vi "Trade.vi"(11 "buffer.in":u64[](array[numeric])=[0, 0, 0, 0, 0, 0, 0, 0, 0]) -> (3 "OrderBook.Command":T1)   [LabVIEW 2020]
doc: "Cboe PITCH Trade (0x2A long, 0x2B short, 0x30 expanded) -> orderbook.command: type Trade (enum value 10, add Trade=10 and Unsupported=11 to orderbook.command.type.ctl), orderId, side, quantity, symbol (8 chars, space padded), price, nanoseconds. Short price keeps 2 implied decimals."
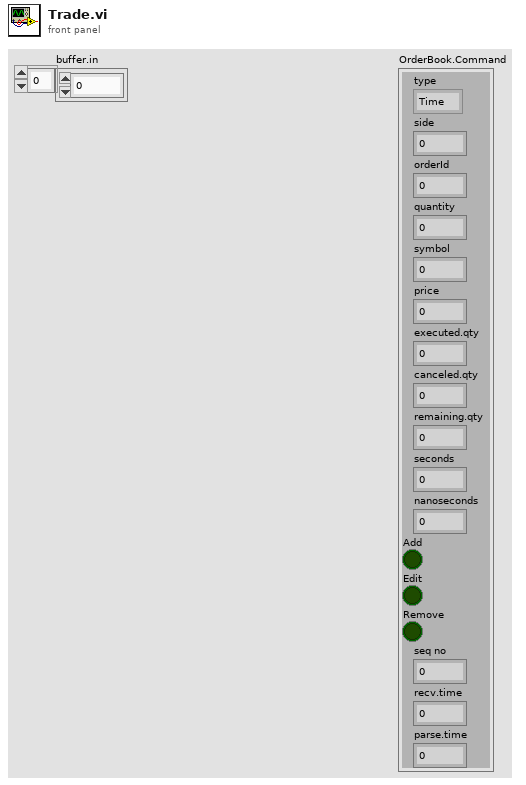
[diagram p1: front panel]
types:
  T1 = cluster{"type":enum8{"Time", "AddOrder", "OrderExecuted", "OrderExecutedAtPrice", "ReduceSize", "ModifyOrder", "DeleteOrder", "Get.Everything", "Get.All.Orders", "Get.Top", "Trade", "Unsupported"}, "side":u8, "orderId ":u64, "quantity":u32, "symbol":u64, "price":u64, "executed.qty":u32, "canceled.qty":u32, "remaining.qty":u32, "seconds":u64, "nanoseconds":u64, "Add":bool, "Edit":bool, "Remove":bool, "seq no":u32, "recv.time":u64, "parse.time":u64}
  T2 = enum8{"Time", "AddOrder", "OrderExecuted", "OrderExecutedAtPrice", "ReduceSize", "ModifyOrder", "DeleteOrder", "Get.Everything", "Get.All.Orders", "Get.Top", "Trade", "Unsupported"}
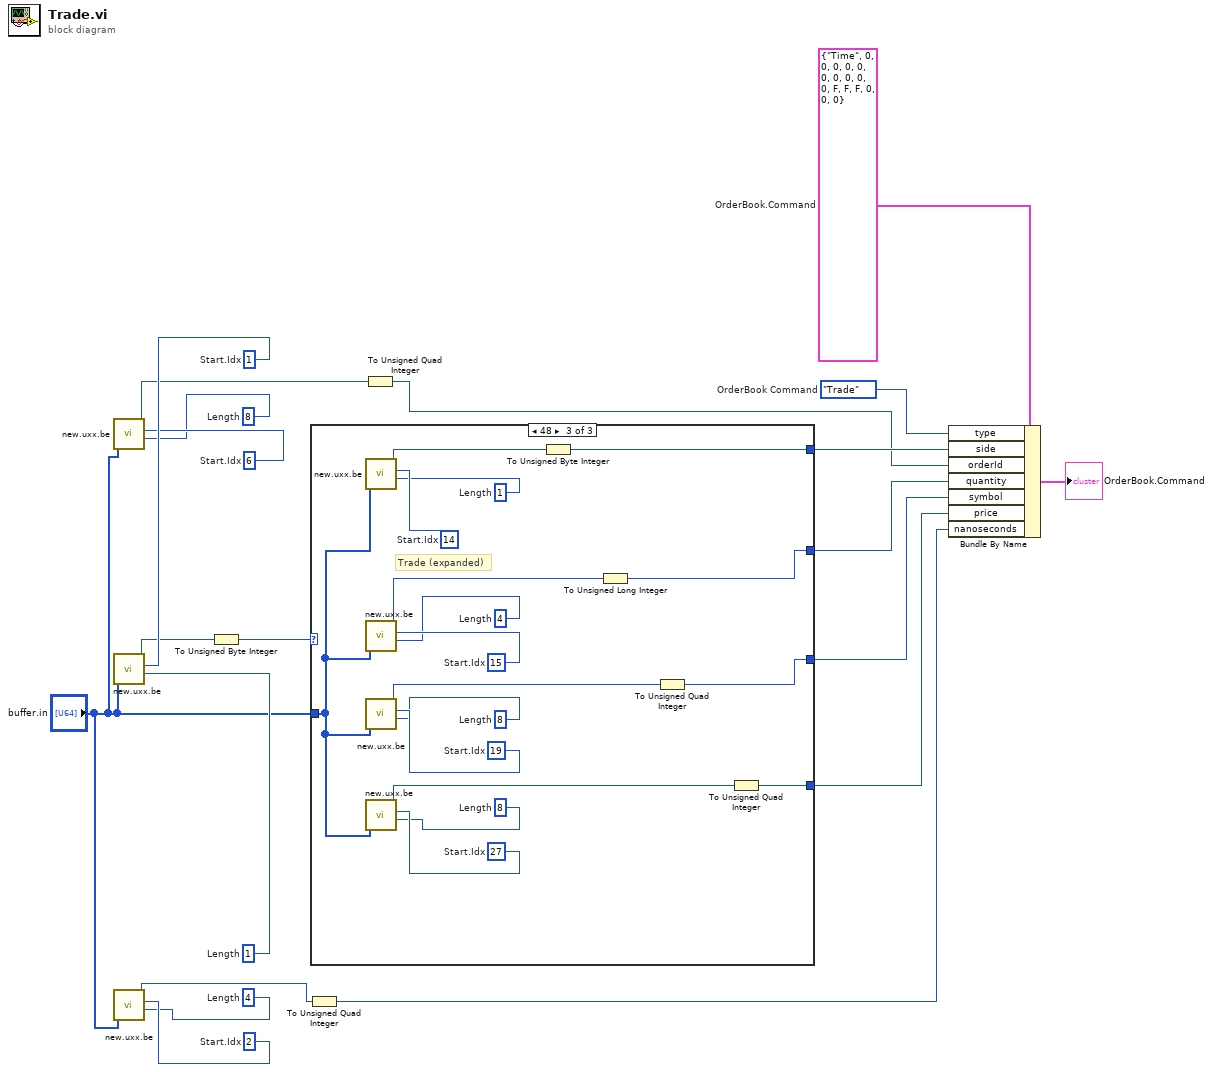
[diagram p0: block diagram]
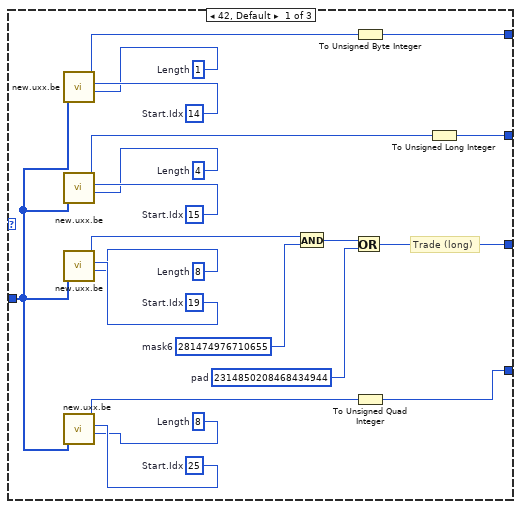
[diagram p2: hidden frame]
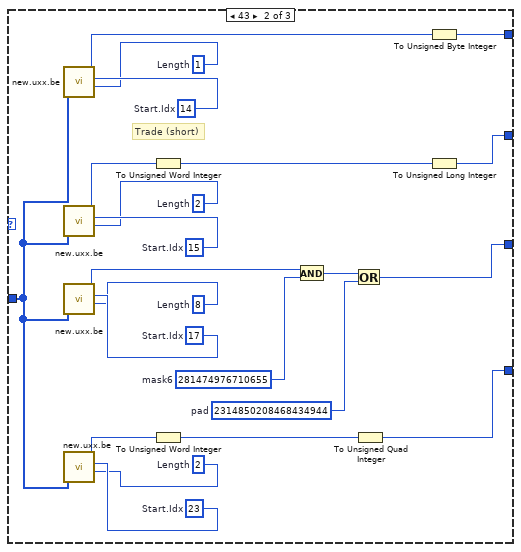
[diagram p3: hidden frame]
diagram:
  w13 = u8 8  # Length
  w14 = u8 6  # Start.Idx
  w16 = u8 4  # Length
  w17 = u8 2  # Start.Idx
  w19 = u8 1  # Length
  w20 = u8 1  # Start.Idx
  w9 = T2."Trade"  # OrderBook Command
  w2 = T1 {"type"=enum."Time", "side"=0, "orderId "=0, "quantity"=0, "symbol"=0, "price"=0, "executed.qty"=0, "canceled.qty"=0, "remaining.qty"=0, "seconds"=0, "nanoseconds"=0, "Add"=FALSE, "Edit"=FALSE, "Remove"=FALSE, "seq no"=0, "recv.time"=0, "parse.time"=0}  # OrderBook.Command
  n1 = call "new.uxx.be.vi"("buffer (U64)"="buffer.in", "Start.Idx"=w14, "Length"=w13) -> ("Out.Value U64"=w12:u64)  [unwired: 7 in]
  n2 = call "new.uxx.be.vi"("buffer (U64)"="buffer.in", "Start.Idx"=w20, "Length"=w19) -> ("Out.Value U64"=w18:u64)  [unwired: 7 in]
  n3 = call "new.uxx.be.vi"("buffer (U64)"="buffer.in", "Start.Idx"=w17, "Length"=w16) -> ("Out.Value U64"=w15:u64)  [unwired: 7 in]
  n4 = To Unsigned Byte Integer(number=w18) -> (unsigned 8bit integer=w10:u8)
  n5 = To Unsigned Quad Integer(1:w15) -> (0:w3:u64)
  n6 = case shown="48" w10 {
    tunnel: "buffer.in" -> [w28 w49 w70]
    tunnel: [w24 w44 w66] -> w8
    tunnel: [w23 w43 w65] -> w6
    tunnel: [w22 w42 w64] -> w5
    tunnel: [w21 w41 w63] -> w4
    frame 42, Default {
      w26 = u8 8  # Length
      w27 = u8 25  # Start.Idx
      w29 = u64 2314850208468434944  # pad
      w31 = u64 281474976710655  # mask6
      w33 = u8 8  # Length
      w34 = u8 19  # Start.Idx
      w36 = u8 4  # Length
      w37 = u8 15  # Start.Idx
      w39 = u8 1  # Length
      w40 = u8 14  # Start.Idx
      # "Trade (long)"
      n7 = call "new.uxx.be.vi"("buffer (U64)"=w28, "Start.Idx"=w40, "Length"=w39) -> ("Out.Value U64"=w38:u64)  [unwired: 7 in]
      n8 = call "new.uxx.be.vi"("buffer (U64)"=w28, "Start.Idx"=w37, "Length"=w36) -> ("Out.Value U64"=w35:u64)  [unwired: 7 in]
      n9 = call "new.uxx.be.vi"("buffer (U64)"=w28, "Start.Idx"=w34, "Length"=w33) -> ("Out.Value U64"=w32:u64)  [unwired: 7 in]
      n10 = call "new.uxx.be.vi"("buffer (U64)"=w28, "Start.Idx"=w27, "Length"=w26) -> ("Out.Value U64"=w25:u64)  [unwired: 7 in]
      n11 = And(x=w32, y=w31) -> (x .and. y?=w30:u64)
      n12 = Or(x=w30, y=w29) -> (x .or. y?=w22:u64)
      n13 = To Unsigned Byte Integer(number=w38) -> (unsigned 8bit integer=w24:u8)
      n14 = To Unsigned Quad Integer(1:w25) -> (0:w21:u64)
      n15 = To Unsigned Long Integer(number=w35) -> (unsigned 32bit integer=w23:u32)
    }
    frame 43 {
      w47 = u8 2  # Length
      w48 = u8 23  # Start.Idx
      w50 = u64 2314850208468434944  # pad
      w52 = u64 281474976710655  # mask6
      w54 = u8 8  # Length
      w55 = u8 17  # Start.Idx
      w58 = u8 2  # Length
      w59 = u8 15  # Start.Idx
      w61 = u8 1  # Length
      w62 = u8 14  # Start.Idx
      # "Trade (short)"
      n16 = call "new.uxx.be.vi"("buffer (U64)"=w49, "Start.Idx"=w62, "Length"=w61) -> ("Out.Value U64"=w60:u64)  [unwired: 7 in]
      n17 = call "new.uxx.be.vi"("buffer (U64)"=w49, "Start.Idx"=w59, "Length"=w58) -> ("Out.Value U64"=w57:u64)  [unwired: 7 in]
      n18 = call "new.uxx.be.vi"("buffer (U64)"=w49, "Start.Idx"=w55, "Length"=w54) -> ("Out.Value U64"=w53:u64)  [unwired: 7 in]
      n19 = call "new.uxx.be.vi"("buffer (U64)"=w49, "Start.Idx"=w48, "Length"=w47) -> ("Out.Value U64"=w46:u64)  [unwired: 7 in]
      n20 = To Unsigned Word Integer(number=w57) -> (unsigned 16bit integer=w56:u16)
      n21 = To Unsigned Word Integer(number=w46) -> (unsigned 16bit integer=w45:u16)
      n22 = And(x=w53, y=w52) -> (x .and. y?=w51:u64)
      n23 = Or(x=w51, y=w50) -> (x .or. y?=w42:u64)
      n24 = To Unsigned Quad Integer(1:w45) -> (0:w41:u64)
      n25 = To Unsigned Byte Integer(number=w60) -> (unsigned 8bit integer=w44:u8)
      n26 = To Unsigned Long Integer(number=w56) -> (unsigned 32bit integer=w43:u32)
    }
    frame 48 {
      w68 = u8 8  # Length
      w69 = u8 27  # Start.Idx
      w72 = u8 8  # Length
      w73 = u8 19  # Start.Idx
      w75 = u8 4  # Length
      w76 = u8 15  # Start.Idx
      w78 = u8 1  # Length
      w79 = u8 14  # Start.Idx
      # "Trade (expanded)"
      n27 = call "new.uxx.be.vi"("buffer (U64)"=w70, "Start.Idx"=w79, "Length"=w78) -> ("Out.Value U64"=w77:u64)  [unwired: 7 in]
      n28 = call "new.uxx.be.vi"("buffer (U64)"=w70, "Start.Idx"=w76, "Length"=w75) -> ("Out.Value U64"=w74:u64)  [unwired: 7 in]
      n29 = call "new.uxx.be.vi"("buffer (U64)"=w70, "Start.Idx"=w73, "Length"=w72) -> ("Out.Value U64"=w71:u64)  [unwired: 7 in]
      n30 = call "new.uxx.be.vi"("buffer (U64)"=w70, "Start.Idx"=w69, "Length"=w68) -> ("Out.Value U64"=w67:u64)  [unwired: 7 in]
      n31 = To Unsigned Byte Integer(number=w77) -> (unsigned 8bit integer=w66:u8)
      n32 = To Unsigned Long Integer(number=w74) -> (unsigned 32bit integer=w65:u32)
      n33 = To Unsigned Quad Integer(1:w71) -> (0:w64:u64)
      n34 = To Unsigned Quad Integer(1:w67) -> (0:w63:u64)
    }
  }
  n35 = To Unsigned Quad Integer(1:w12) -> (0:w7:u64)
  n36 = Bundle By Name(cluster=w2, "type"=w9, "side"=w8, "orderId"=w7, "quantity"=w6, "symbol"=w5, "price"=w4, "nanoseconds"=w3) -> (→"OrderBook.Command":T1)
